vi "SR830 set sin out voltage.vi"(8 "error in (no error)":errorcluster, 10 "voltage":dbl[unit], 11 "VISA resource name":refnum<visa-resource-name>) -> (0 "error out":errorcluster, 3 "VISA resource name out":refnum<visa-resource-name>)   [LabVIEW 2009, in "Lockin.lvclass"]
doc: "Sets the voltage of the SINE OUT output of the lock-in amplifier."
uses:
  Lockin.lvclass
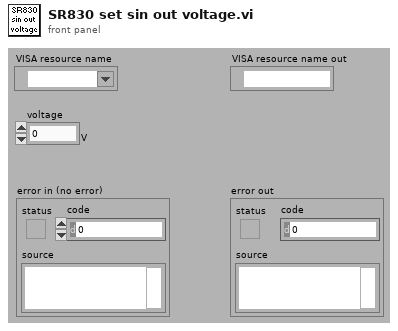
[diagram p1: front panel]
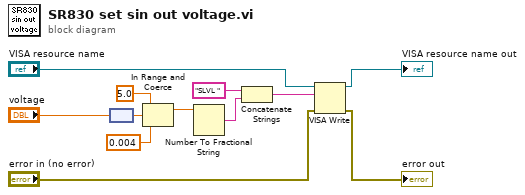
[diagram p0: block diagram]
diagram:
  n1 = node("voltage") -> (w1:dbl)
  n2 = In Range and Coerce(upper limit=5.0, x=w1, lower limit=0.004) -> (coerced(x)=w12:dbl)  [unwired: 1 out]
  n3 = Number To Fractional String(number=w12) -> (F-format string=w8:string)  [unwired: 3 out]
  n4 = Concatenate Strings("SLVL " ("write buffer"), w8) -> (w6:string)
  n5 = VISA Write(VISA resource name="VISA resource name", write buffer=w6, error in (no error)="error in (no error)") -> (VISA resource name out=→"VISA resource name out":refnum<visa-resource-name>, error out=→"error out":errorcluster)  [unwired: 1 out]
